vi "start_photon_stream.vi"(8 "error in (no error)":errorcluster, 11 "hydraharp in":refnum<class "hydraharp.lvclass">) -> (0 "error out":errorcluster, 3 "hydraharp out":refnum<class "hydraharp.lvclass">)   [LabVIEW 2015, in "hydraharp.lvclass"]
uses:
  hydraharp.lvclass
  hydraharp.lvclass/hydraharp.ctl
  hydraharp_fifo_queue_data.ctl
  hydraharp_fifo_actions.ctl
  hhlib.dll
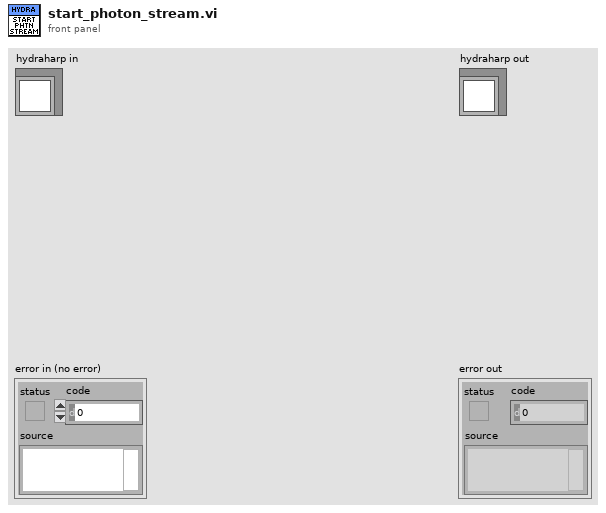
[diagram p1: front panel]
types:
  T1 = typedef "hydraharp_fifo_queue_data.ctl" = cluster{"fifo_buffer":u32[], "fifo_action":T2}
  T2 = typedef "hydraharp_fifo_actions.ctl" = enum16{"stop", "new_data"}
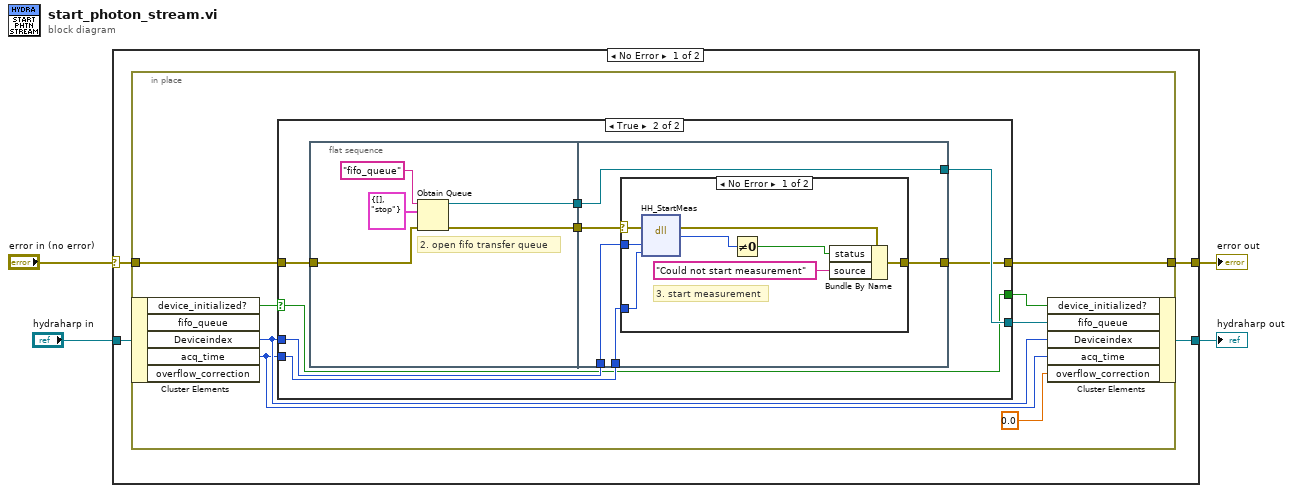
[diagram p0: block diagram]
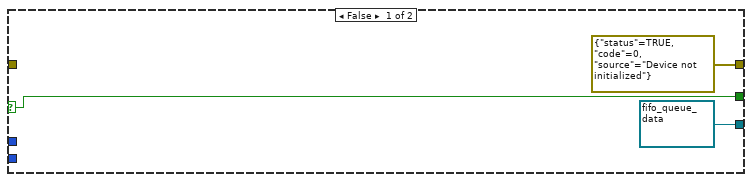
[diagram p2: hidden frame]
diagram:
  n1 = case shown="No Error" "error in (no error)" {
    selector: "error in (no error)" -> [w5 w47]
    tunnel: "hydraharp in" -> [w8 w48]
    tunnel: [w7 w47] -> w2
    tunnel: [w6 w48] -> w1
    frame No Error {
      n2 = in-place {
        in-place-border: [w13] -> w7
        in-place-border: w5 -> [w9]
        n3 = in-place-cluster #1(w8) -> ("device_initialized?"=w16:bool, "Deviceindex"=w12:i32, "acq_time"=w11:i32)  [unwired: 2 out]
        n4 = case shown="True" w16 {
          selector: w16 -> [w17 w21]
          tunnel: [refnum<queue> refnum ("queue out") w25] -> w14
          tunnel: w11 -> [_ w24]
          tunnel: [errorcluster {"status"=TRUE, "code"=0, "source"="Device not initialized"} ("error IO") w23] -> w13
          tunnel: w12 -> [_ w22]
          tunnel: [w17 w21] -> w15
          tunnel: w9 -> [_ w20]
          frame False {
          }
          frame True {
            n5 = flat-sequence {
              tunnel: [w30] -> w27
              tunnel: [w29] -> w26
              tunnel: w20 -> [w28]
              tunnel: [w37] -> w25
              tunnel: w27 -> [w33]
              tunnel: w26 -> [w37]
              tunnel: w24 -> [w36]
              tunnel: [w35] -> w23
              tunnel: w22 -> [w34]
              frame #0 {
                # "2. open fifo transfer queue"
                n6 = Obtain Queue(name (unnamed)="fifo_queue", element data type=T1 {"fifo_buffer"=[], "fifo_action"=enum."stop"} ("fifo_queue_data"), error in (no error)=w28) -> (queue out=w29:refnum<queue>, error out=w30:errorcluster)  [unwired: 2 in, 1 out]
              }
              frame #1 {
                n7 = case shown="No Error" w33 {
                  selector: w33 -> [w38 w46]
                  tunnel: w36 -> [w45 _]
                  tunnel: [w40 w46] -> w35
                  tunnel: w34 -> [w39 _]
                  frame No Error {
                    # "3. start measurement"
                    n8 = dll-call lib="hhlib.dll" fn="HH_StartMeas"(error in=w38, "devidx"=w39, "tacq"=w45) -> (error out=w43:errorcluster, w44:i32)  [unwired: 4 in, 1 out]
                    n9 = Not Equal To 0?(x=w44) -> (x != 0?=w42:bool)
                    n10 = Bundle By Name(cluster=w43, "status"=w42, "source"="Could not start measurement") -> (w40:errorcluster)
                  }
                  frame Error {
                  }
                }
              }
            }
          }
        }
        n11 = in-place-cluster #1("device_initialized?"=w15, "fifo_queue"=w14, "Deviceindex"=w12, "acq_time"=w11, "overflow_correction"=0.0) -> (w6:refnum<class "hydraharp.lvclass">)
      }
    }
    frame Error {
    }
  }
  "error out" <- w2
  "hydraharp out" <- w1
